vi "GDSLvIcon_CalculateBrightness.vi"(11 "RGB Color In":u32(colorbox)) -> (1 "SuggestedTextColor":u32(colorbox), 2 "BrightColor(Use Black text for better contrast)":bool, 3 "BrightnessValue":dbl)   [LabVIEW 2020]
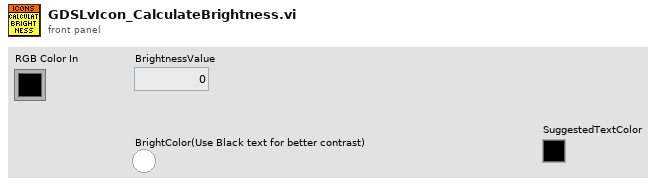
[diagram p1: front panel]
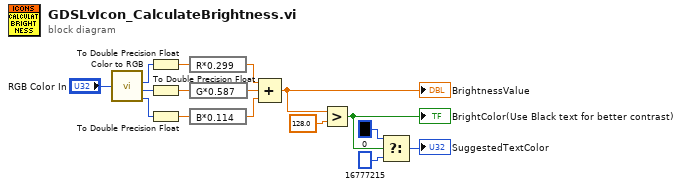
[diagram p0: block diagram]
diagram:
  n1 = call <vilib>:"Color to RGB.vi"("Color"="RGB Color In") -> ("R"=w9:u8, "G"=w10:u8, "B"=w11:u8)  [unwired: 1 out]
  n2 = To Double Precision Float(number=w9) -> (double precision float=w14:dbl)
  n3 = To Double Precision Float(number=w10) -> (double precision float=w13:dbl)
  n4 = To Double Precision Float(number=w11) -> (double precision float=w12:dbl)
  n5 = expression code="R*0.299"(w14) -> (w7:dbl)
  n6 = expression code="G*0.587"(w13) -> (w6:dbl)
  n7 = expression code="B*0.114"(w12) -> (w8:dbl)
  n8 = Compound Arithmetic op=ADD(w7, w6, w8) -> (w15:dbl)
  "BrightnessValue" <- w15
  n9 = Greater?(x=w15, y=128.0) -> (0:w2:bool)
  "BrightColor(Use Black text for better contrast)" <- w2
  n10 = Select(t=u32 0, s=w2, f=u32 16777215) -> (s? t:f=→"SuggestedTextColor":u32)
